vi "Frame Update Data From Script.vi"(8 "error in (no error)":errorcluster, 10 "Frame Number":u32, 11 "IDE simple in":refnum<class "Main Panel.lvclass">) -> (0 "error out":errorcluster, 3 "IDE simple out":refnum<class "Main Panel.lvclass">)   [LabVIEW 2018, in "Main Panel.lvlib" / "Main Panel.lvclass"]
uses:
  Main Panel.lvclass
  Main Panel.lvclass/Main Panel.ctl
  Frame Analizer/Data Parser.lvclass
  ScintillaNET/ScintillaNET.lvclass
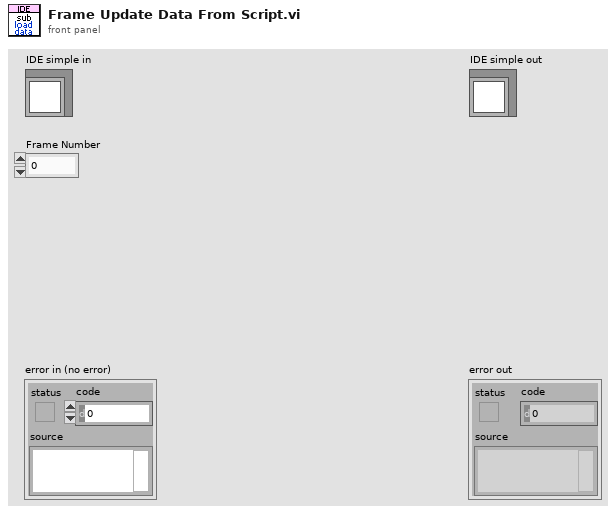
[diagram p1: front panel]
types:
  T1 = typedef "Data Parser.lvclass/frame data.ctl" = cluster{"Title":T2, "Basic Data":T3, "Sound":string, "<o> Data":T4, "<bp> Data":T5, "<c> Data":T6, "<w> Data":T7, "<i> Data Array":T8[], "<b> Data Array":T9[]}
  T2 = typedef "Data Parser.lvclass/frame title.ctl" = cluster{"Number":string, "Name":string}
  T3 = typedef "Data Parser.lvclass/frame basic data.ctl" = cluster{"Basic":cluster{"pic":string, "state":string, "wait":string, "next":string}, "Move":cluster{"dvx":string, "dvy":string, "dvz":string}, "Pic Center":cluster{"centerx":string, "centery":string}, "Skill":cluster{"hit_a":string, "hit_d":string, "hit_j":string, "hit_Fa":string, "hit_Ua":string, "hit_Da":string, "hit_Fj":string, "hit_Uj":string, "hit_Dj":string, "hit_ja":string}, "Mp":string}
  T4 = typedef "Data Parser.lvclass/frame o data.ctl" = cluster{"kind":string, "x":string, "y":string, "action":string, "dvx":string, "dvy":string, "dvz":string, "oid":string, "facing":string}
  T5 = typedef "Data Parser.lvclass/frame bp data.ctl" = cluster{"x":string, "y":string}
  T6 = typedef "Data Parser.lvclass/frame c data.ctl" = cluster{"kind":string, "x":string, "y":string, "injury":string, "cover":string, "vaction":string, "aaction":string, "taction":string, "hurtable":string, "decrease":string, "fronthurtact":string, "backhurtact":string, "dircontrol":string, "throwvx":string, "throwvy":string, "throwvz":string, "throwinjury":string}
  T7 = typedef "Data Parser.lvclass/frame w data.ctl" = cluster{"kind":string, "x":string, "y":string, "weaponact":string, "dvx":string, "dvy":string, "dvz":string, "attacking":string, "cover":string}
  T8 = typedef "Data Parser.lvclass/frame i data.ctl" = cluster{"kind":string, "x":string, "y":string, "w":string, "h":string, "dvx":string, "dvy":string, "dvz":string, "fall":string, "arest":string, "vrest":string, "bdefend":string, "injury":string, "zwidth":string, "effect":string, "catchingact":string, "caughtact":string}
  T9 = typedef "Data Parser.lvclass/frame b data.ctl" = cluster{"kind":string, "x":string, "y":string, "w":string, "h":string}
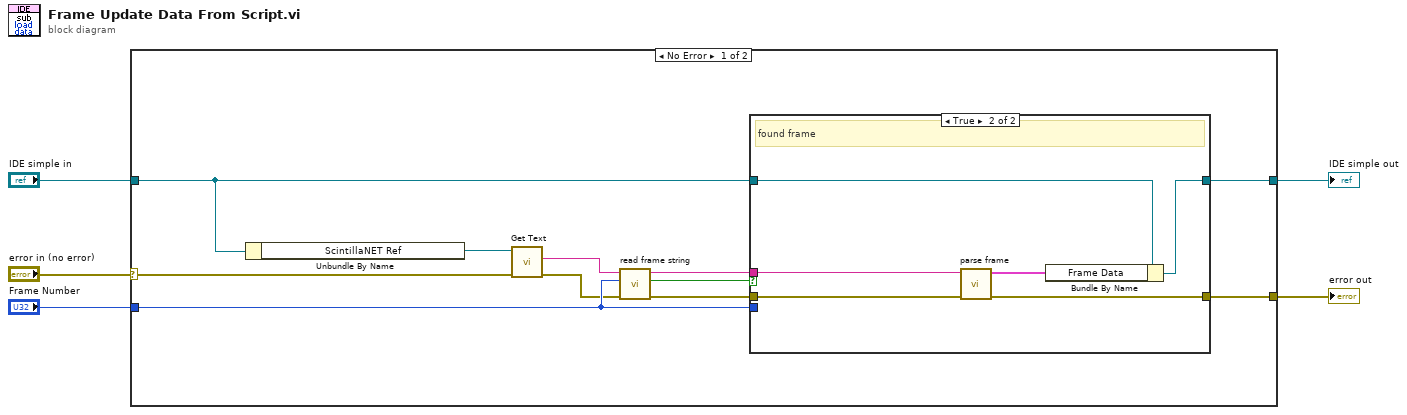
[diagram p0: block diagram]
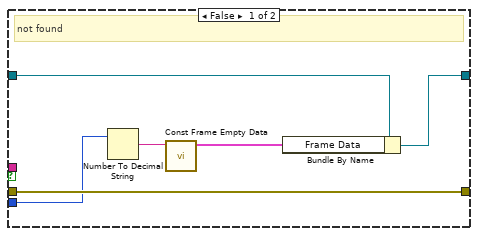
[diagram p2: hidden frame]
diagram:
  n1 = case shown="No Error" "error in (no error)" {
    selector: "error in (no error)" -> [w8 w30]
    tunnel: [w11 w30] -> w4
    tunnel: [w12 w29] -> w2
    tunnel: "IDE simple in" -> [w14 w29]
    tunnel: "Frame Number" -> [w10 _]
    frame No Error {
      n2 = Unbundle By Name(w14) -> ("ScintillaNET Ref"=w9:refnum<class "ScintillaNET.lvclass">)
      n3 = call "Get Text.vi"("error in (no error)"=w8, "ScintillaNET in"=w9) -> ("error out"=w6:errorcluster, "Text"=w7:string)  [unwired: 7 in, 1 out]
      n4 = call "read frame string.vi"("error in"=w6, "frame number"=w10, "file string"=w7) -> ("error out"=w15:errorcluster, "found"=w13:bool, "<f> string"=w16:string)  [unwired: 5 in, 1 out]
      n5 = case shown="True" w13 {
        tunnel: w16 -> [_ w28]
        tunnel: w15 -> [w21 w27]
        tunnel: w14 -> [w22 w26]
        tunnel: [w21 w23] -> w11
        tunnel: [w20 w24] -> w12
        tunnel: w10 -> [w18 _]
        frame False {
          # "not found"
          n6 = Number To Decimal String(number=w18) -> (decimal integer string=w17:string)  [unwired: 1 in]
          n7 = call "Const Frame Empty Data.vi"("frame number"=w17) -> ("frame data"=w19:T1)  [unwired: 10 in]
          n8 = Bundle By Name(cluster=w22, "Frame Data"=w19) -> (w20:refnum<class "Main Panel.lvclass">)
        }
        frame True {
          # "found frame"
          n9 = call "parse frame.vi"("error in (no error)"=w27, "<f> string"=w28) -> ("error out"=w23:errorcluster, "frame data"=w25:T1)  [unwired: 8 in]
          n10 = Bundle By Name(cluster=w26, "Frame Data"=w25) -> (w24:refnum<class "Main Panel.lvclass">)
        }
      }
    }
    frame Error {
    }
  }
  "error out" <- w4
  "IDE simple out" <- w2
